vi "LJcounterUD.vi"() -> ()   [LabVIEW 2021]
panel:
  in  "Write On Change":bool
  in  "Data File":path=path "c:/temp/data.dat"
  in  "Write To File":bool
  in  "Reset Counter":bool=TRUE
  in  "Measurement Type":u16(ring) items=["Frequency", "Count"]
  out "Measurement":dbl format="%.2f"
  out "Error Message":string
  in  "stop":bool
  in  "Interval (seconds)":dbl=1.0 min=0.025 format="%.2f"
  # "www.labjack.com"
  # "Uses the first found U3 or UE9 over USB.  Counter appears on FIO0 on the UE9, and\nFIO4 on the U3.  Uses a hardware counter."
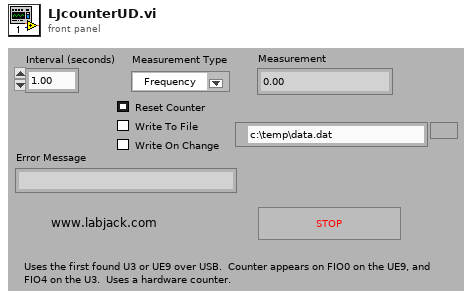
[diagram p1: front panel]
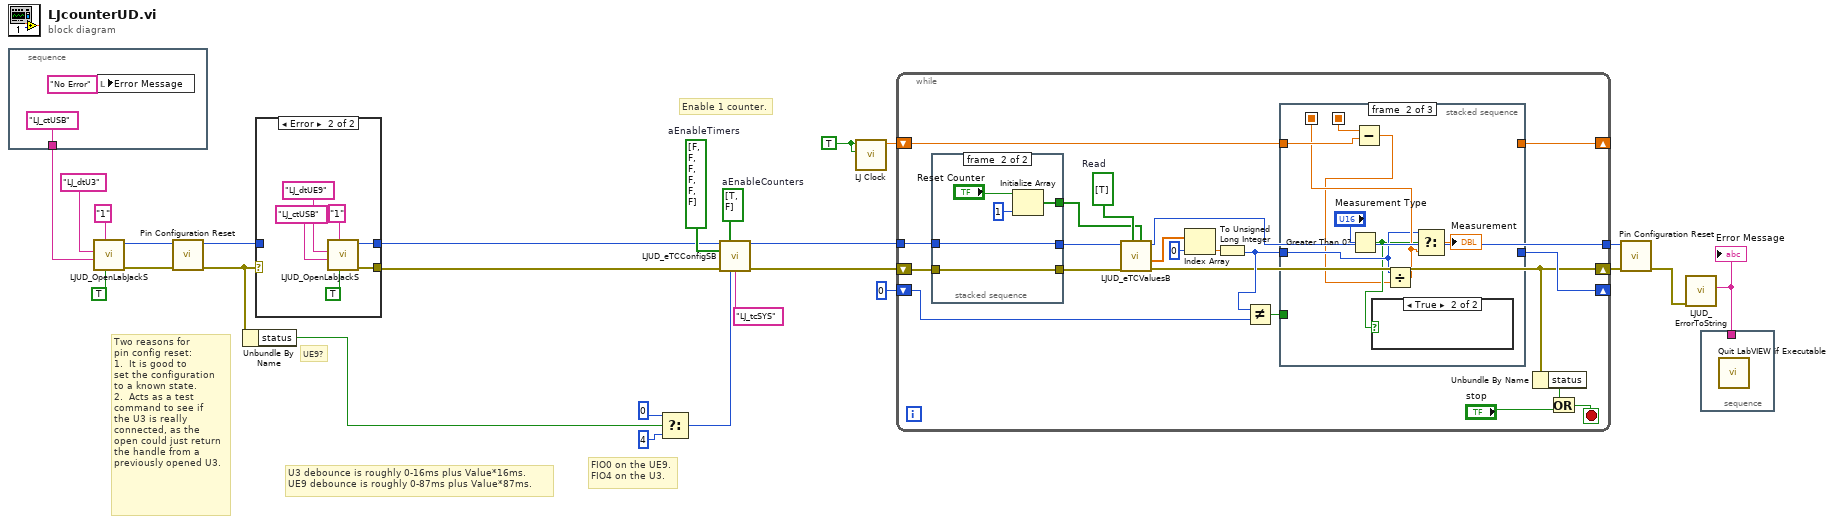
[diagram p0: block diagram]
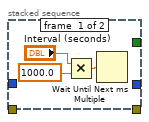
[diagram p2: hidden frame]
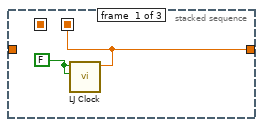
[diagram p3: hidden frame]
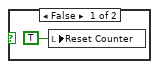
[diagram p4: hidden frame]
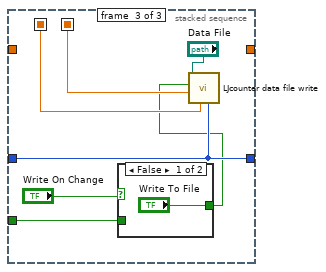
[diagram p5: hidden frame]
diagram:
  w22 = bool[] [TRUE, FALSE]  # aEnableCounters
  w23 = bool[] [FALSE, FALSE, FALSE, FALSE, FALSE, FALSE]  # aEnableTimers
  w26 = TRUE ("Initialize")
  # "U3 debounce is roughly 0-16ms plus Value*16ms.\nUE9 debounce is roughly 0-87ms plus Value*87ms."
  # "FIO0 on the UE9.\nFIO4 on the U3."
  # "Two reasons for\npin config reset:\n1.  It is good to\nset the configuration\nto a known state.\n2.  Acts as a test\ncommand to see if\nthe U3 is really\nconnected, as the\nopen could just return\nthe handle from a\npreviously opened U3."
  # "UE9?"
  # "Enable 1 counter."
  n1 = stacked-sequence {
    tunnel: ["LJ_ctUSB" ("ConnectionType")] -> w14
    frame #0 {
      n2 = local write "Error Message"("No Error" ("Error Message")) -> ()
    }
  }
  n3 = call "LJUD_OpenLabJackS.vi"("FirstFound"=TRUE, "Address"="1", "ConnectionType"=w14, "DeviceType"="LJ_dtU3") -> ("error out"=w10:errorcluster, "Handle"=w11:i32)  [unwired: 5 in, 1 out]
  n4 = call "Pin Configuration Reset.vi"("error in"=w10, "Handle In"=w11) -> ("error out"=w9:errorcluster, "Handle Out"=w8:i32)  [unwired: 8 in]
  n5 = Unbundle By Name(w9) -> ("status"=w3:bool)
  n6 = case shown="Error" w9 {
    selector: w9 -> [w29 _]
    tunnel: [w29 w32] -> w6
    tunnel: [w30 w31] -> w7
    tunnel: w8 -> [w30 _]
    frame No Error {
    }
    frame Error {
      n7 = call "LJUD_OpenLabJackS.vi"("FirstFound"=TRUE, "Address"="1", "ConnectionType"="LJ_ctUSB", "DeviceType"="LJ_dtUE9") -> ("error out"=w32:errorcluster, "Handle"=w31:i32)  [unwired: 5 in, 1 out]
    }
  }
  n8 = Select(t=0 ("TCPinOffset"), s=w3, f=4) -> (s? t:f=w4:i32)
  n9 = call "LJUD_eTCConfigSB.vi"("Handle In"=w7, "aEnableCounters"=w22, "aEnableTimers"=w23, "error in"=w6, "TCPinOffset"=w4, "TimerClockBase"="LJ_tcSYS") -> ("Handle Out"=w20:i32, "error out"=w21:errorcluster)  [unwired: 8 in]
  n10 = call "LJ Clock.vi"("Sync to second"=w26, "Initialize"=w26) -> ("Seconds since 1/1/1904 universal time"=w25:ext)  [unwired: 9 in]
  n11 = while {
    tunnel: [w40] -> w16
    tunnel: w20 -> [w49]
    shift-left: w21 -> [w52]
    shift-right: [w44] -> w18
    shift-left: u32 0 -> [w45]
    shift-right: [w53] -> _
    shift-left: w25 -> [w55]
    shift-right: [w56] -> _
    stop <- w41 stop-if-true
    w39 = bool[] [TRUE]  # Read
    n12 = stacked-sequence {
      tunnel: w52 -> [_ w64]
      tunnel: [_ w64] -> w51
      tunnel: [_ w63] -> w50
      tunnel: w49 -> [_ w63]
      tunnel: [_ w60] -> w38
      frame #0 {
        n13 = Multiply(x="Interval (seconds)", y=1000.0) -> (x*y=w58:dbl)
        n14 = Wait Until Next ms Multiple(millisecond multiple=w58) -> ()  [unwired: 1 out]
      }
      frame #1 {
        n15 = Initialize Array("Reset Counter", 1 ("Dimension Size")) -> (w60:bool[])
      }
    }
    n16 = call "LJUD_eTCValuesB.vi"("aResetCounters"=w38, "aReadCounters"=w39, "error in"=w51, "Handle In"=w50) -> ("error out"=w44:errorcluster, "aCounterValues"=w37:dbl[], "Handle Out"=w40:i32)  [unwired: 4 in, 1 out]
    n17 = Index Array(array=w37, index=0 ("Index")) -> (element=w47:dbl)
    n18 = To Unsigned Long Integer(number=w47) -> (unsigned 32bit integer=w46:u32)
    n19 = Not Equal?(x=w46, y=w45) -> (x != y?=w54:bool)
    n20 = stacked-sequence {
      seq-local: [w65 _ _] -> [_ w72 w81]
      seq-local: [_ w70 _] -> [_ _ w80]
      tunnel: w46 -> [_ w69 w77]
      tunnel: [w65 _ _] -> w56
      tunnel: w55 -> [_ w71 _]
      tunnel: w54 -> [_ _ w78]
      tunnel: [_ _ w77] -> w53
      frame #0 {
        w66 = FALSE ("Initialize")
        n21 = call "LJ Clock.vi"("Sync to second"=w66, "Initialize"=w66) -> ("Seconds since 1/1/1904 universal time"=w65:ext)  [unwired: 9 in]
      }
      frame #1 {
        n22 = Greater Than 0?(x="Measurement Type") -> (x > 0?=w68:bool)
        n23 = Subtract(x=w72, y=w71) -> (x-y=w67:ext)
        n24 = case shown="True" w68 {
          frame False {
            n25 = local write "Reset Counter"(TRUE ("Reset Counter")) -> ()
          }
          frame True {
          }
        }
        n26 = Divide(x=w69, y=w67) -> (x/y=w70:ext)
        n27 = Select(t=w69, s=w68, f=w70) -> (s? t:f=→"Measurement":ext)
      }
      frame #2 {
        n28 = case shown="False" "Write On Change" {
          tunnel: w78 -> [_ w84]
          tunnel: ["Write To File" w84] -> w76
          frame False {
          }
          frame True {
          }
        }
        n29 = call "LJcounter data file write.vi"("Count"=w77, "Frequency"=w80, "seconds"=w81, "Write To File"=w76, "Data File"="Data File") -> ()  [unwired: 6 in, 1 out]
      }
    }
    n30 = Unbundle By Name(w44) -> ("status"=w43:bool)
    n31 = Or(x=w43, y="stop") -> (x .or. y?=w41:bool)
  }
  n32 = call "Pin Configuration Reset.vi"("error in"=w18, "Handle In"=w16) -> ("error out"=w19:errorcluster)  [unwired: 8 in, 1 out]
  n33 = call "LJUD_ErrorToString.vi"("error in"=w19) -> ("String"=w17:string)  [unwired: 10 in]
  "Error Message" <- w17
  n34 = stacked-sequence {
    tunnel: w17 -> [_]
    frame #0 {
      n35 = call "Quit LabVIEW if Executable.vi"() -> ()  [unwired: 1 in]
    }
  }
